vi "Motor Control Message Loop.vi"(8 "error in (no error)":errorcluster, 11 "Message Queues":T1) -> (0 "error out":errorcluster)   [LabVIEW 2016, in "Motor Control.lvlib"]
doc: "The message loop subVI to handle messages pertaining to logging data."
uses:
  Motor Control.lvlib
  support/Message Queue/All Message Queues.ctl
  support/Message Queue/Message Cluster.ctl
  Motor Control State.ctl
  Motor Control Config.ctl
  Speed and Duration.ctl
  support/Message Queue/Enqueue Message (Single).vi
  <vilib>/Utility/error.llb/Error Cluster From Error Code.vi
  <vilib>/ErrorRing/Error Ring.xnode
  support/Message Queue/Message Queue.lvlib
  <instrlib>/Pololu Motor Controller/Pololu Motor Controller.lvlib
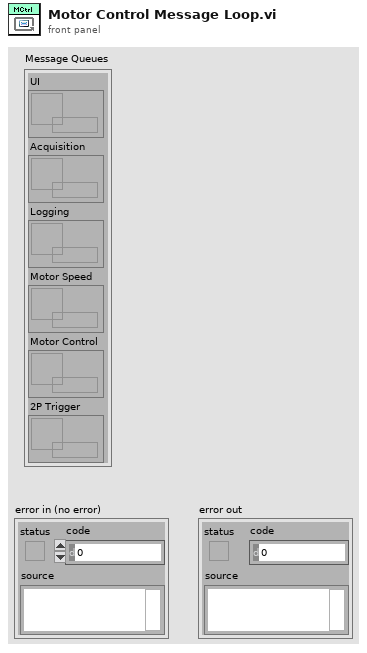
[diagram p1: front panel]
types:
  T1 = typedef "Message Queue.lvlib/All Message Queues.ctl" = cluster{"UI":refnum<queue>, "Acquisition":refnum<queue>, "Logging":refnum<queue>, "Motor Speed":refnum<queue>, "Motor Control":refnum<queue>, "2P Trigger":refnum<queue>}
  T2 = typedef "Motor Control.lvlib/Motor Control State.ctl" = enum16{"Idle", "Running"}
  T3 = typedef "Motor Control.lvlib/Motor Control Config.ctl" = cluster{"VISA resource name":refnum<visa-resource-name>, "Speed and Duration":T4[]}
  T4 = typedef "Motor Control.lvlib/Speed and Duration.ctl" = cluster{"Speed (%)":i32, "Duration (sec)":dbl}
  T5 = cluster{"Baud Rate":u32, "Parity":u16, "Data Bits":u16, "Stop Bits":u16, "Flow Control":u16}
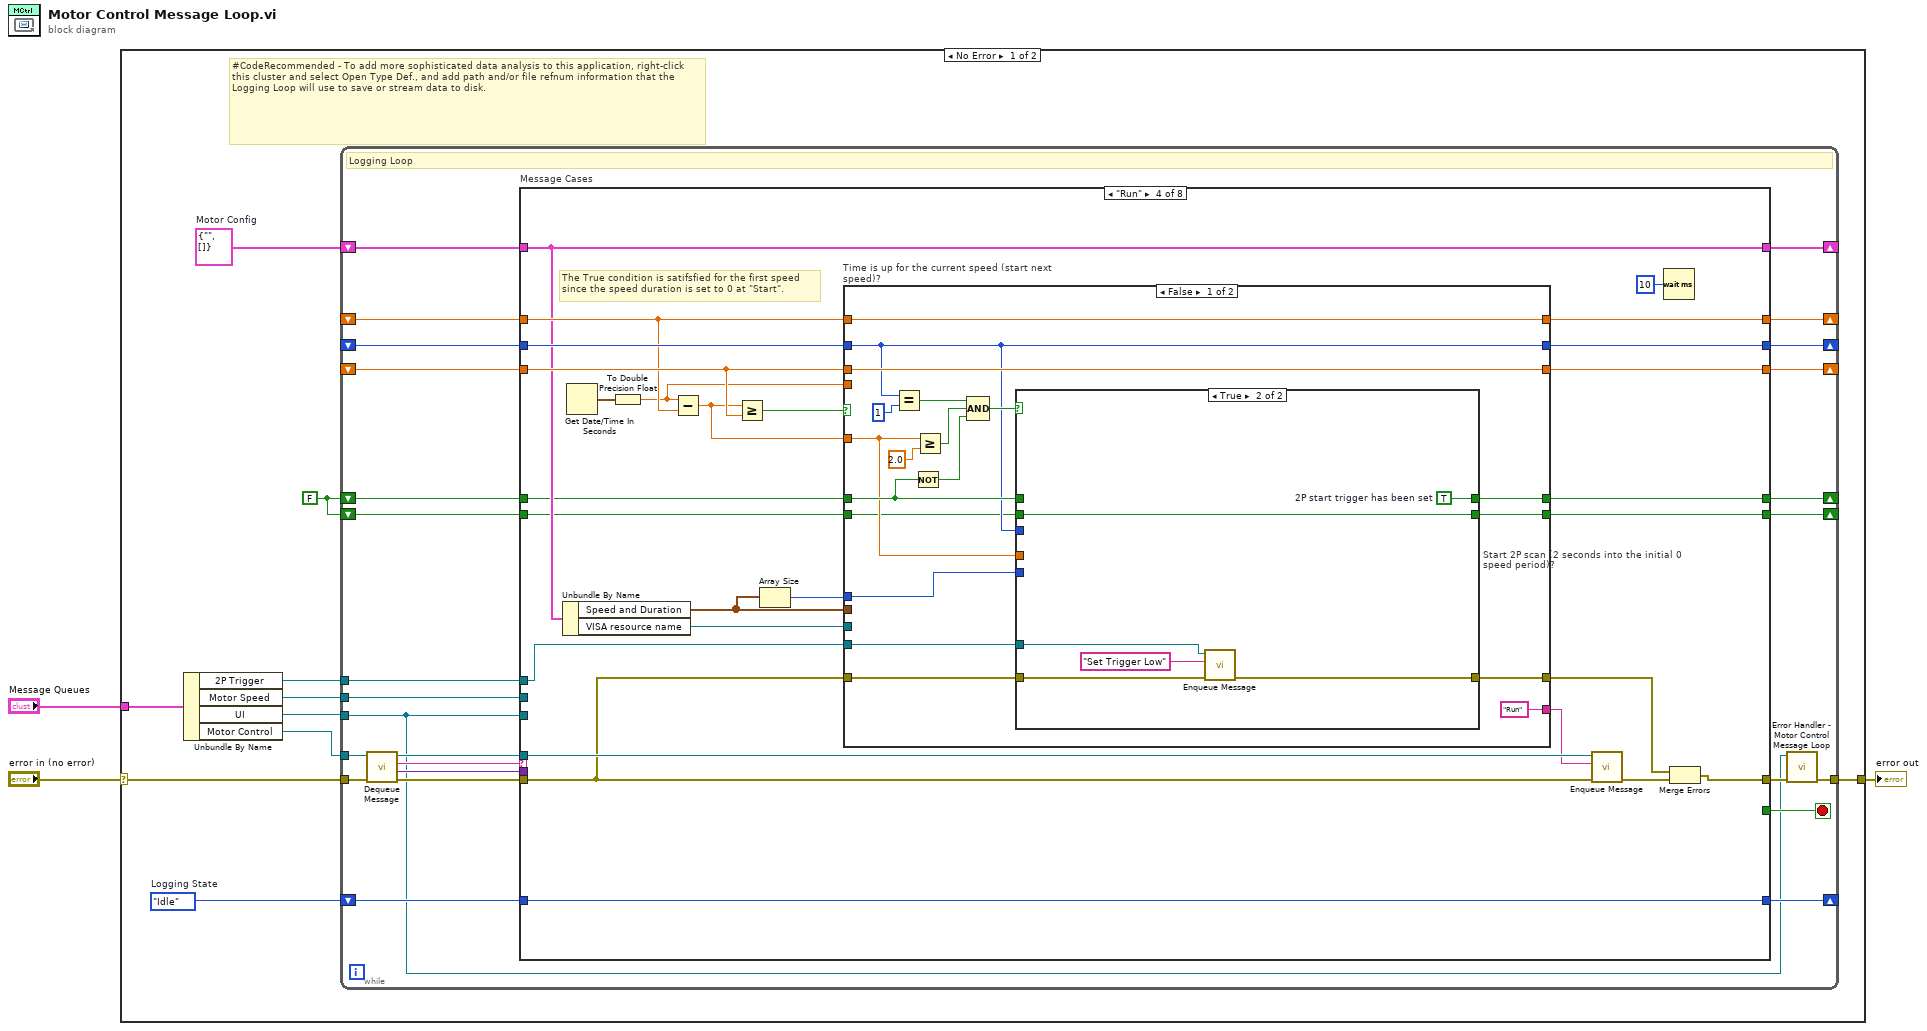
[diagram p0: block diagram]
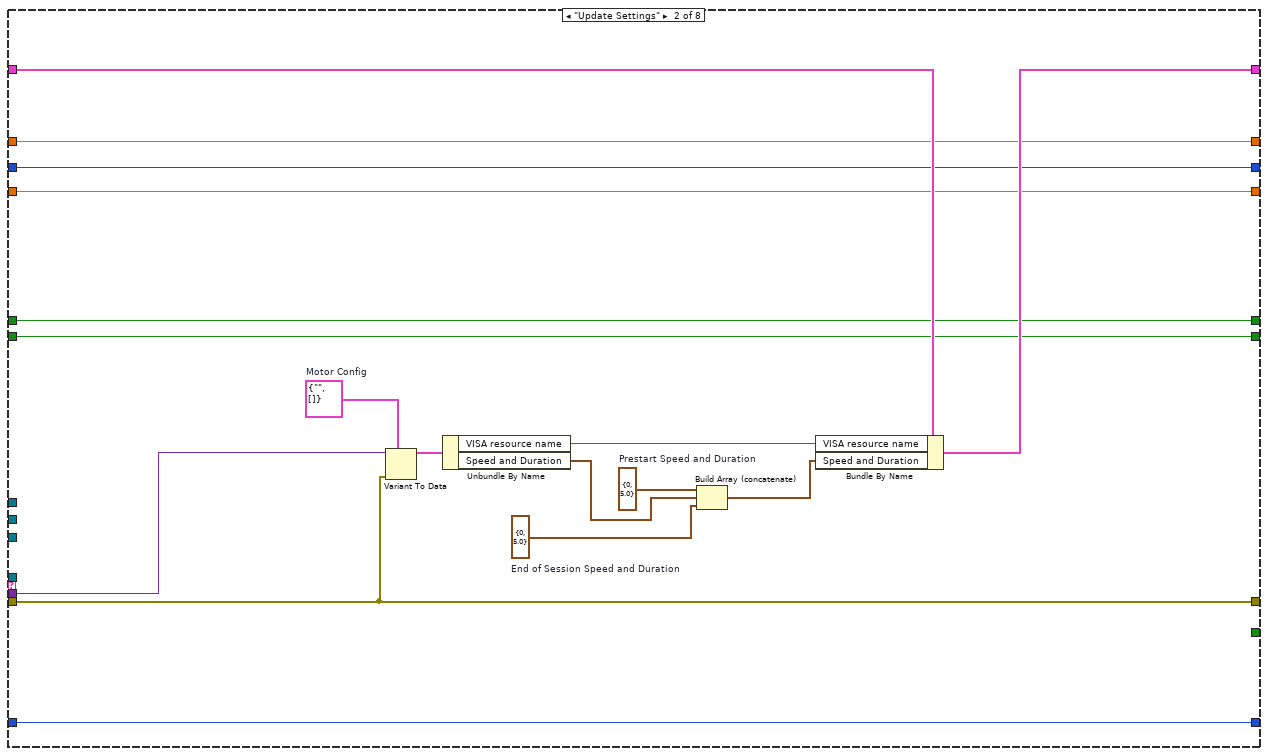
[diagram p3: hidden frame]
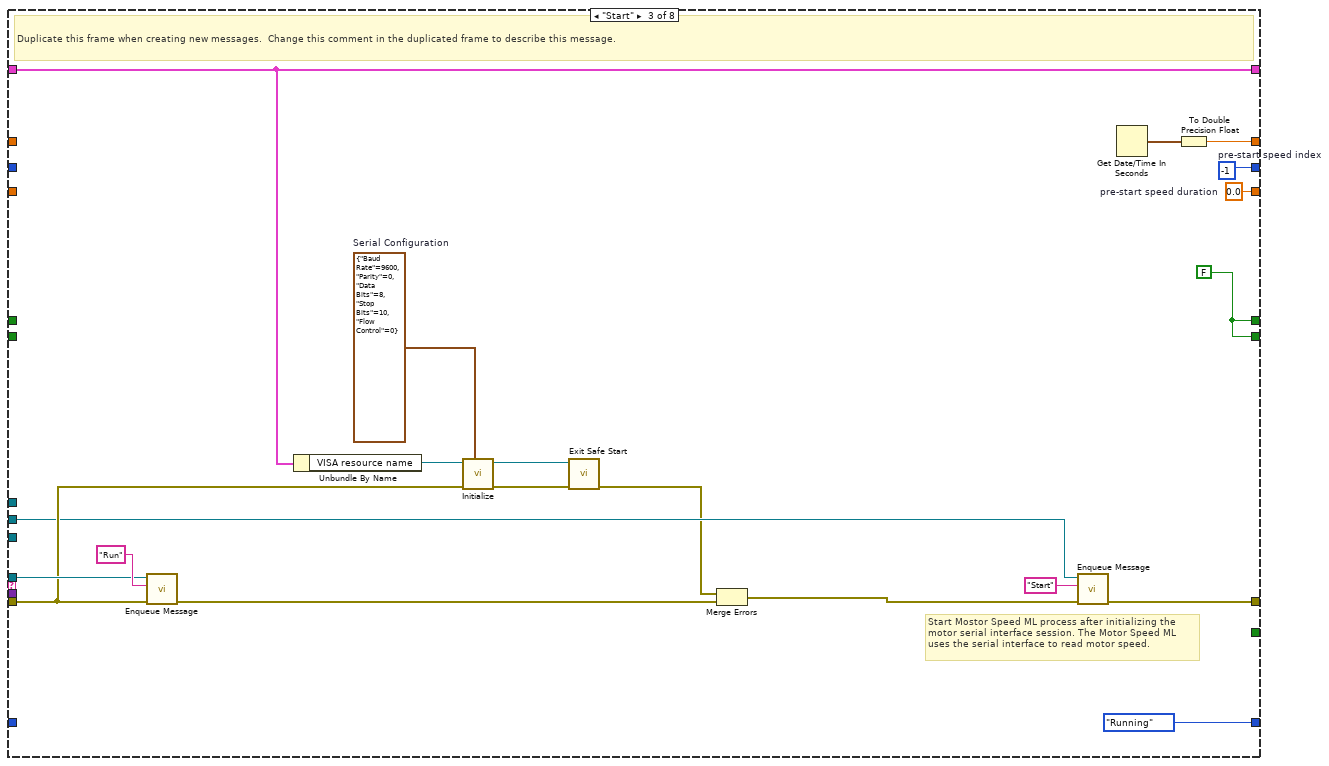
[diagram p4: hidden frame]
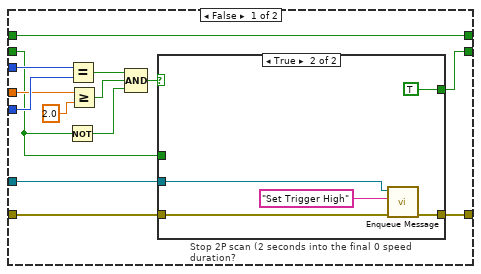
[diagram p5: hidden frame]
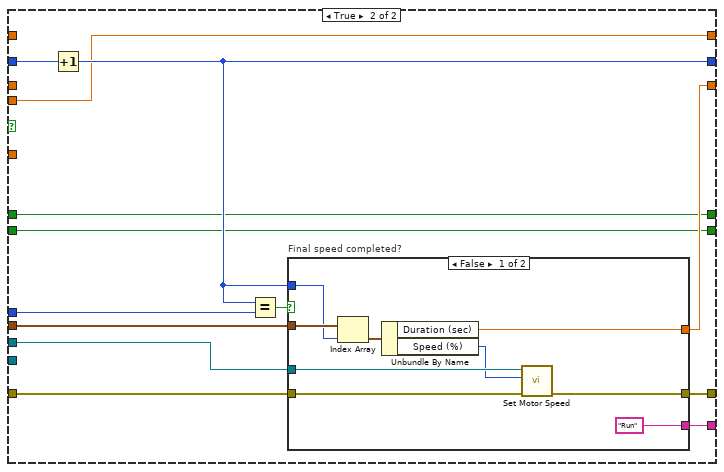
[diagram p7: hidden frame]
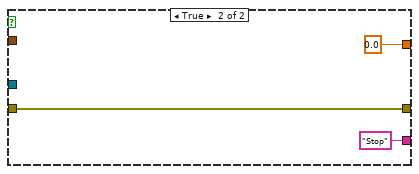
[diagram p8: hidden frame]
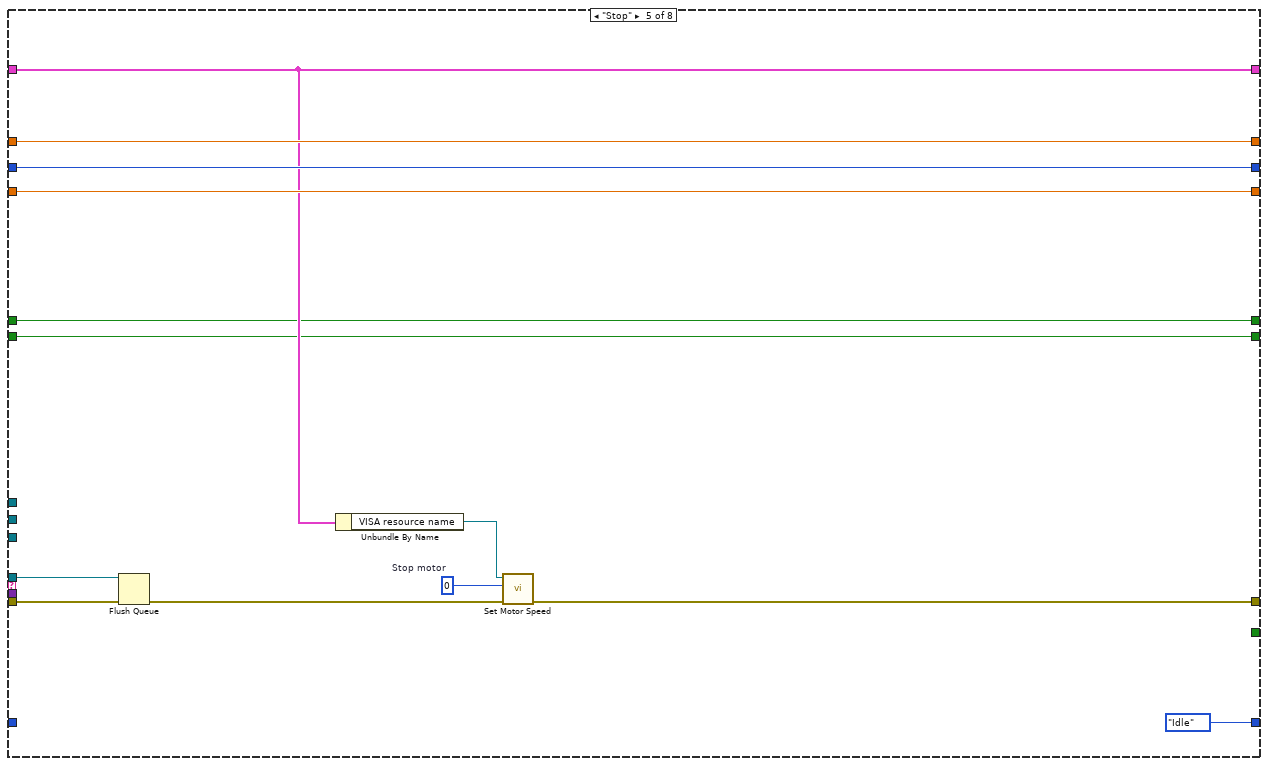
[diagram p9: hidden frame]
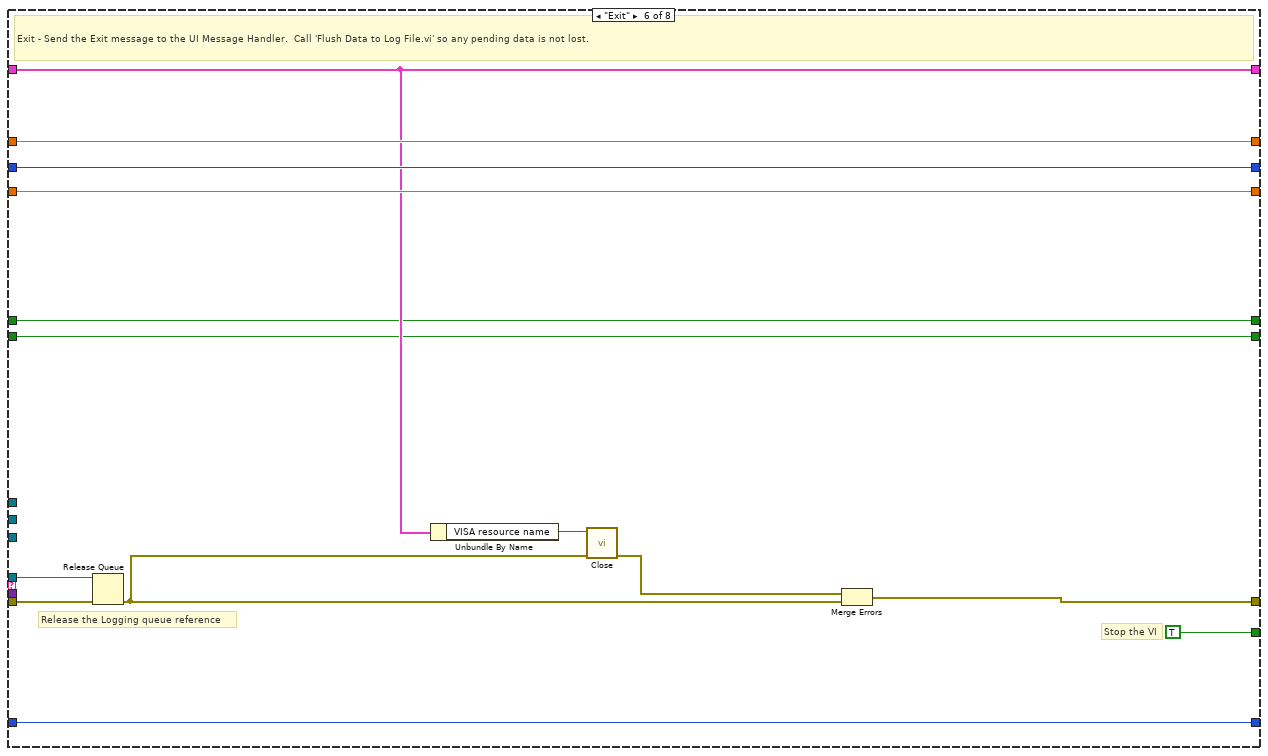
[diagram p10: hidden frame]
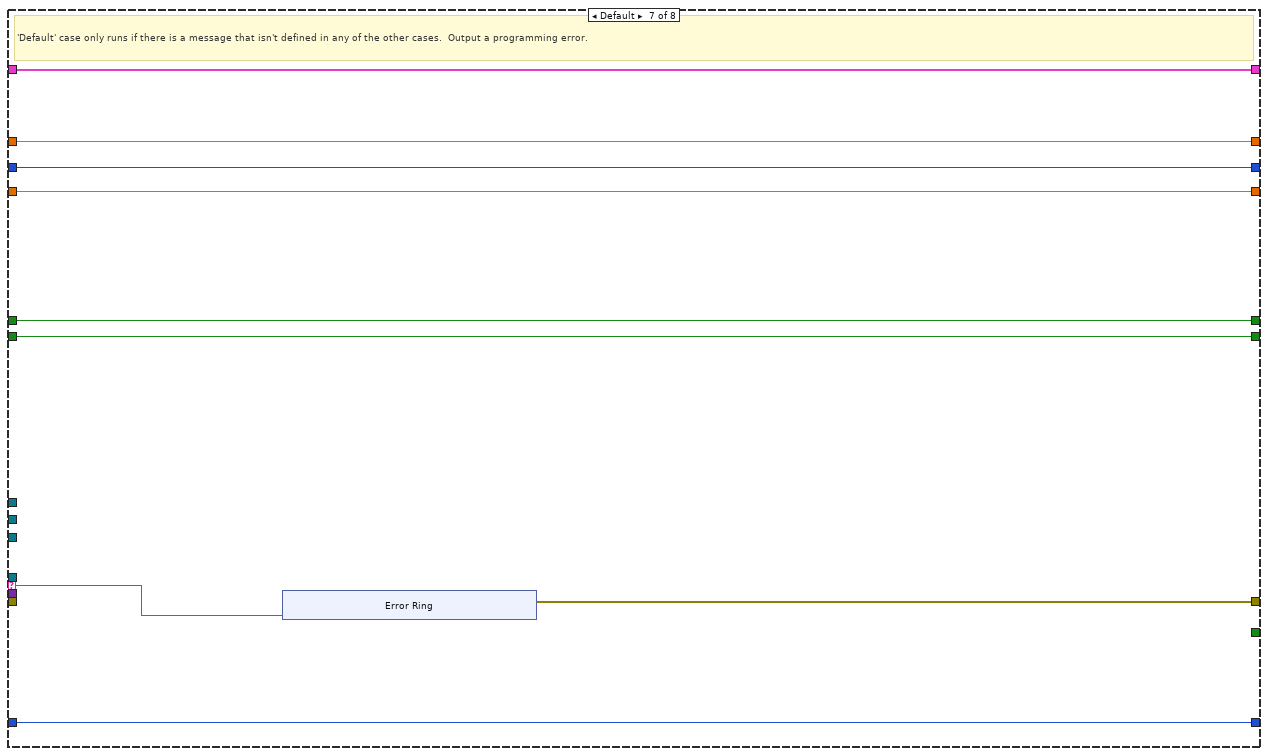
[diagram p11: hidden frame]
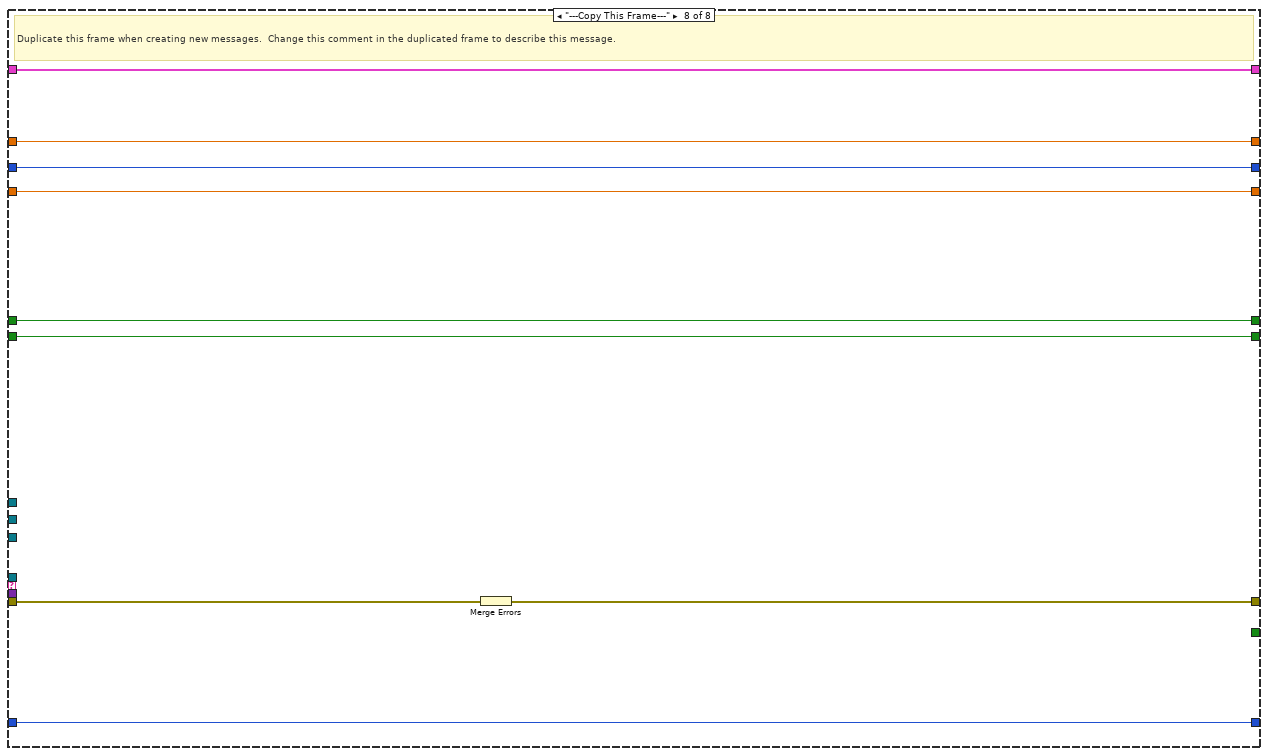
[diagram p12: hidden frame]
diagram:
  n1 = case shown="No Error" "error in (no error)" {
    selector: "error in (no error)" -> [w10 w235]
    tunnel: "Message Queues" -> [w13 _]
    tunnel: [w11 w235] -> w2
    frame No Error {
      w4 = FALSE
      w7 = T3 {"VISA resource name"="", "Speed and Duration"=[]}  # Motor Config
      w8 = Motor_Control_State."Idle"  # Logging State
      # "#CodeRecommended - To add more sophisticated data analysis to this application, right-click this cluster and select Open Type Def., and add path and/or file refnum information that the Logging Loop will use to save or stream data to disk."
      n2 = Unbundle By Name(w13) -> ("2P Trigger"=w5:refnum<queue>, "Motor Speed"=w6:refnum<queue>, "UI"=w9:refnum<queue>, "Motor Control"=w12:refnum<queue>)
      n3 = while {
        tunnel: w12 -> [w31]
        shift-right: [w38] -> _
        shift-left: w7 -> [w39]
        tunnel: w9 -> [w26]
        shift-right: [w29] -> _
        shift-left: w8 -> [w30]
        tunnel: w10 -> [w36]
        tunnel: [w28] -> w11
        shift-right: [w25] -> _
        shift-left: _ -> [w24]
        shift-right: [w23] -> _
        shift-left: _ -> [w22]
        shift-right: [w21] -> _
        shift-left: _ -> [w20]
        tunnel: w6 -> [w19]
        shift-right: [w16] -> _
        shift-left: w4 -> [w18]
        shift-right: [w15] -> _
        shift-left: w4 -> [w17]
        tunnel: w5 -> [w14]
        stop <- w37 stop-if-true
        # "Logging Loop"
        n4 = call "Dequeue Message.vi"("error in (no error)"=w36, "Message Queue"=w31) -> ("error out"=w35:errorcluster, "Message Data"=w33:variant, "Message"=w34:string, "dup Message Queue"=w32:refnum<queue>)  [unwired: 6 in]
        n5 = case "Message Cases" shown="\"Run\"" w34 {
          selector: w34 -> [_ _ _ _ _ _ w215 _]
          tunnel: w32 -> [_ _ w83 w110 w194 w206 _ _]
          tunnel: w35 -> [w46 w63 w77 w102 w195 w207 _ w234]
          tunnel: [w46 w63 w70 w109 w188 w208 w216 w232] -> w27
          tunnel: w39 -> [w47 w61 w76 w93 w187 w199 w218 w233]
          tunnel: [w47 w60 w76 w93 w187 w199 w218 w233] -> w38
          tunnel: [_ _ _ _ _ TRUE _ _] -> w37
          tunnel: w33 -> [_ w62 _ _ _ _ _ _]
          tunnel: w26 -> [_ _ _ _ _ _ _ _]
          tunnel: w30 -> [w45 w64 _ w111 _ w205 w217 w231]
          tunnel: [w45 w64 Motor_Control_State."Running" ("Logging State") w111 Motor_Control_State."Idle" ("Logging State") w205 w217 w231] -> w29
          tunnel: [w44 w56 w80 w98 w192 w204 w214 w230] -> w25
          tunnel: w24 -> [w44 w56 _ w97 w192 w204 w214 w230]
          tunnel: [w43 w55 w79 w106 w191 w203 w213 w229] -> w23
          tunnel: w22 -> [w43 w55 _ w105 w191 w203 w213 w229]
          tunnel: [w42 w54 w78 w104 w190 w202 w212 w228] -> w21
          tunnel: w20 -> [w42 w54 _ w103 w190 w202 w212 w228]
          tunnel: w19 -> [_ _ w71 _ _ _ _ _]
          tunnel: w18 -> [w41 w49 _ w89 w184 w197 w211 w227]
          tunnel: w17 -> [w40 w48 _ w86 w183 w196 w210 w226]
          tunnel: [w41 w49 w65 w87 w184 w197 w211 w227] -> w16
          tunnel: [w40 w48 w65 w85 w183 w196 w210 w226] -> w15
          tunnel: w14 -> [_ _ _ w88 _ _ _ _]
          frame "Initialize" {
            # "Initialize - gets called when first launched. Currently a no-op."
          }
          frame "Update Settings" {
            w51 = T4 {"Speed (%)"=0, "Duration (sec)"=5.0}  # End of Session Speed and Duration
            w53 = T4 {"Speed (%)"=0, "Duration (sec)"=5.0}  # Prestart Speed and Duration
            w57 = T3 {"VISA resource name"="", "Speed and Duration"=[]}  # Motor Config
            n6 = Variant To Data(error in=w63, type=w57, Variant=w62) -> (data=w58:T3)  [unwired: 1 out]
            n7 = Unbundle By Name(w58) -> ("VISA resource name"=w59:refnum<visa-resource-name>, "Speed and Duration"=w52:T4[])
            n8 = Build Array (concatenate)(w53, w52, w51) -> (w50:T4[])
            n9 = Bundle By Name(cluster=w61, "VISA resource name"=w59, "Speed and Duration"=w50) -> (w60:T3)
          }
          frame "Start" {
            w65 = FALSE
            w73 = T5 {"Baud Rate"=9600, "Parity"=0, "Data Bits"=8, "Stop Bits"=10, "Flow Control"=0}  # Serial Configuration
            w78 = 0.0  # pre-start speed duration
            w79 = -1  # pre-start speed index
            # "Start Mostor Speed ML process after initializing the\nmotor serial interface session. The Motor Speed ML\nuses the serial interface to read motor speed."
            # "Duplicate this frame when creating new messages.  Change this comment in the duplicated frame to describe this message."
            n10 = call-poly "Enqueue Message.vi"("error in (no error)"=w77, "Message"="Run", "Message Queue"=w83) -> ("error out"=w74:errorcluster)  [unwired: 7 in, 1 out]
            n11 = Unbundle By Name(w76) -> ("VISA resource name"=w75:refnum<visa-resource-name>)
            n12 = call <instrlib>:"Initialize.vi"("Serial Configuration"=w73, "error in (no error)"=w77, "VISA resource name"=w75) -> ("error out"=w68:errorcluster, "VISA resource name out"=w66:refnum<visa-resource-name>)  [unwired: 5 in, 2 out]
            n13 = call <instrlib>:"Exit Safe Start.vi"("error in (no error)"=w68, "VISA resource name"=w66) -> ("error out"=w67:errorcluster)  [unwired: 7 in, 2 out]
            n14 = Merge Errors(w67, w74) -> (w69:errorcluster)
            n15 = call-poly "Enqueue Message.vi"("error in (no error)"=w69, "Message"="Start", "Message Queue"=w71) -> ("error out"=w70:errorcluster)  [unwired: 7 in, 1 out]
            n16 = Get Date/Time In Seconds() -> (seconds since 1Jan1904=w81:timestamp)
            n17 = To Double Precision Float(number=w81) -> (double precision float=w80:dbl)
          }
          frame "Run" {
            # "The True condition is satifsfied for the first speed\nsince the speed duration is set to 0 at \"Start\"."
            n18 = Unbundle By Name(w93) -> ("Speed and Duration"=w92:T4[], "VISA resource name"=w94:refnum<visa-resource-name>)
            n19 = Get Date/Time In Seconds() -> (seconds since 1Jan1904=w107:timestamp)
            n20 = To Double Precision Float(number=w107) -> (double precision float=w95:dbl)
            n21 = Subtract(x=w95, y=w97) -> (x-y=w90:dbl)
            n22 = Greater Or Equal?(x=w90, y=w103) -> (x >= y?=w100:bool)
            n23 = Array Size(array=w92) -> (size(s)=w91:i32)
            n24 = case "Time is up for the current speed (start next speed)?" shown="False" w100 {
              tunnel: w105 -> [w116 w170]
              tunnel: [w116 w164] -> w106
              tunnel: [w130 w169] -> w104
              tunnel: w103 -> [w130 _]
              tunnel: w102 -> [w127 w166]
              tunnel: [w126 w167] -> w101
              tunnel: ["Run" ("Message") w165] -> w99
              tunnel: [w128 w163] -> w98
              tunnel: w97 -> [w128 _]
              tunnel: w95 -> [_ w163]
              tunnel: w92 -> [_ w162]
              tunnel: w94 -> [_ w161]
              tunnel: w91 -> [w115 w160]
              tunnel: w90 -> [w114 _]
              tunnel: w89 -> [w117 w159]
              tunnel: w88 -> [w119 _]
              tunnel: [w118 w159] -> w87
              tunnel: w86 -> [w113 w158]
              tunnel: [w112 w158] -> w85
              frame False {
                n25 = Equal?(x=w116, y=1) -> (x = y?=w123:bool)
                n26 = Not(x=w117) -> (.not. x?=w121:bool)
                n27 = Greater Or Equal?(x=w114, y=2.0) -> (x >= y?=w122:bool)
                n28 = Compound Arithmetic op=AND(w123, w122, w121) -> (w120:bool)
                n29 = case "Start 2P scan (2 seconds into the initial 0 speed period)?" shown="True" w120 {
                  tunnel: w127 -> [w137 w156]
                  tunnel: [w138 w155] -> w126
                  tunnel: w119 -> [w133 w154]
                  tunnel: [w144 w153] -> w118
                  tunnel: w117 -> [w144 _]
                  tunnel: w116 -> [w139 _]
                  tunnel: w115 -> [w136 _]
                  tunnel: w114 -> [w135 _]
                  tunnel: w113 -> [w131 w152]
                  tunnel: [w132 w152] -> w112
                  frame False {
                    n30 = Not(x=w131) -> (.not. x?=w140:bool)
                    n31 = Equal?(x=w139, y=w136) -> (x = y?=w142:bool)
                    n32 = Greater Or Equal?(x=w135, y=2.0) -> (x >= y?=w141:bool)
                    n33 = Compound Arithmetic op=AND(w142, w141, w140) -> (w134:bool)
                    n34 = case "Stop 2P scan (2 seconds into the final 0 speed duration?" shown="True" w134 {
                      tunnel: [w146 w150] -> w138
                      tunnel: w137 -> [w146 w151]
                      tunnel: w133 -> [_ w149]
                      tunnel: [w145 TRUE] -> w132
                      tunnel: w131 -> [w145 _]
                      frame False {
                      }
                      frame True {
                        n35 = call-poly "Enqueue Message.vi"("error in (no error)"=w151, "Message"="Set Trigger High", "Message Queue"=w149) -> ("error out"=w150:errorcluster)  [unwired: 7 in, 1 out]
                      }
                    }
                  }
                  frame True {
                    w153 = TRUE  # 2P start trigger has been set
                    n36 = call-poly "Enqueue Message.vi"("error in (no error)"=w156, "Message"="Set Trigger Low", "Message Queue"=w154) -> ("error out"=w155:errorcluster)  [unwired: 7 in, 1 out]
                  }
                }
              }
              frame True {
                n37 = Increment(x=w170) -> (x+1=w164:i32)
                n38 = Equal?(x=w164, y=w160) -> (x = y?=w168:bool)
                n39 = case "Final speed completed?" shown="False" w168 {
                  tunnel: w162 -> [w177 _]
                  tunnel: [w178 0.0 ("Duration (sec)")] -> w169
                  tunnel: w164 -> [w176 _]
                  tunnel: [w173 w182] -> w167
                  tunnel: w166 -> [w174 w182]
                  tunnel: ["Run" ("Message") "Stop" ("Message")] -> w165
                  tunnel: w161 -> [w172 _]
                  frame False {
                    n40 = Index Array(array=w177, index=w176) -> (element=w179:T4)
                    n41 = Unbundle By Name(w179) -> ("Duration (sec)"=w178:dbl, "Speed (%)"=w171:i32)
                    n42 = call <instrlib>:"Set Motor Speed.vi"("error in (no error)"=w174, "Speed (%)"=w171, "VISA resource name"=w172) -> ("error out"=w173:errorcluster)  [unwired: 7 in, 1 out]
                  }
                  frame True {
                  }
                }
              }
            }
            n43 = call-poly "Enqueue Message.vi"("error in (no error)"=w102, "Message"=w99, "Message Queue"=w110) -> ("error out"=w108:errorcluster)  [unwired: 7 in, 1 out]
            n44 = Wait (ms)(milliseconds to wait=u32 10) -> ()  [unwired: 1 out]
            n45 = Merge Errors(w101, w108) -> (w109:errorcluster)
          }
          frame "Stop" {
            w185 = 0  # Stop motor
            n46 = Flush Queue(queue=w194, error in (no error)=w195) -> (error out=w189:errorcluster)  [unwired: 2 out]
            n47 = Unbundle By Name(w187) -> ("VISA resource name"=w186:refnum<visa-resource-name>)
            n48 = call <instrlib>:"Set Motor Speed.vi"("error in (no error)"=w189, "Speed (%)"=w185, "VISA resource name"=w186) -> ("error out"=w188:errorcluster)  [unwired: 7 in, 1 out]
          }
          frame "Exit" {
            # "Release the Logging queue reference"
            # "Stop the VI"
            # "Exit - Send the Exit message to the UI Message Handler.  Call 'Flush Data to Log File.vi' so any pending data is not lost."
            n49 = Release Queue(queue=w206, error in (no error)=w207) -> (error out=w201:errorcluster)  [unwired: 1 in, 2 out]
            n50 = Unbundle By Name(w199) -> ("VISA resource name"=w198:refnum<visa-resource-name>)
            n51 = call <instrlib>:"Close.vi"("error in (no error)"=w201, "VISA resource name"=w198) -> ("error out"=w200:errorcluster)  [unwired: 9 in]
            n52 = Merge Errors(w200, w201) -> (w208:errorcluster)
          }
          frame Default {
            # "'Default' case only runs if there is a message that isn't defined in any of the other cases.  Output a programming error."
            n53 = xnode "Error Ring"("parameter 0"=w215) -> ("error out"=w216:errorcluster)
          }
          frame "---Copy This Frame---" {
            # "Duplicate this frame when creating new messages.  Change this comment in the duplicated frame to describe this message."
            n54 = Merge Errors(w234) -> (w232:errorcluster)
          }
        }
        n55 = call "Error Handler - Motor Control Message Loop.vi"("error in (no error)"=w27, "Message Queue"=w26) -> ("dup error in"=w28:errorcluster)  [unwired: 8 in, 1 out]
      }
    }
    frame Error {
    }
  }
  "error out" <- w2
